vi "NI VeriStand - Get Property Names List.vi"(8 "error in (no error)":errorcluster, 11 "Item Ref in":T1 format="%.0x") -> (0 "error out":errorcluster, 2 "Property Names":string[](array[string]), 3 "Item Ref out":T1 format="%.0x")   [LabVIEW 2020, in "Custom Device Offline API.lvlib"]
uses:
  <vilib>/NI VeriStand/Custom Device Offline API/Custom Device Offline API.lvlib
  <vilib>/NI VeriStand/Custom Device API/Custom Device Item Ref.ctl
  NationalInstruments.VeriStand.SystemDefinitionAPI
  <vilib>/NI VeriStand/Custom Device API/Custom Device API.lvlib
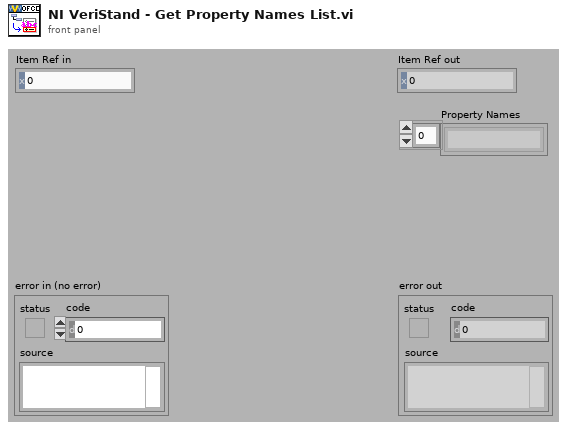
[diagram p1: front panel]
types:
  T1 = typedef "Custom Device API.lvlib/Custom Device Item Ref.ctl" = u64
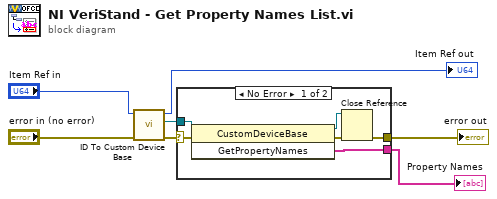
[diagram p0: block diagram]
diagram:
  n1 = call <vilib>:"ID To Custom Device Base.vi"("error in (no error)"="error in (no error)", "ID in"="Item Ref in") -> ("error out"=w4:errorcluster, "BaseNode"=w3:refnum<k24>, "ID out"=→"Item Ref out":u64)  [unwired: 7 in]
  n2 = case shown="No Error" w4 {
    selector: w4 -> [w12 w14]
    tunnel: w3 -> [w13 _]
    tunnel: [w9 w14] -> w2
    tunnel: [w8 _] -> w1
    frame No Error {
      n3 = invoke class="CustomDeviceBase" method="GetPropertyNames"(reference=w13, error in=w12) -> (reference out=w10:refnum<k24>, error out=w11:errorcluster, "GetPropertyNames"=w8:string[])  [unwired: 1 in]
      n4 = Close Reference(reference=w10, error in (no error)=w11) -> (error out=w9:errorcluster)
    }
    frame Error {
    }
  }
  "error out" <- w2
  "Property Names" <- w1
